vi "Autonomous Independent.vi"() -> ()   [LabVIEW 2020]
doc: "This VI is called when autonomous begins, and will automatically be terminated when autonomous ends. You can carry out timed or sensor driven robot movement independently without needing to return to the caller."
uses:
  <vilib>/Rock Robotics/Network Tables/NT Read String.vi
  <vilib>/Rock Robotics/WPI/Utilities/WPI_GetSetVariantRefNum.vi
  <vilib>/Rock Robotics/WPI/RobotDrive/WPI_RobotDriveArcadeDrive_Standard(NoSaturation).vi
  <vilib>/Rock Robotics/Network Tables/NT Write Numeric Array.vi
panel:
  out "Current Movement, for debugging":T1 {"Y Joystick Value" scale=1.0..-1.0; "X Joystick Value" scale=-1.0..1.0}
  in  "Array of robot movements":T2(array[cluster])=[{"X Joystick Value"=0.39393939393939403, "Y Joystick Value"=0.0, "Delay (sec)"=1.0, "Movement Name"="turn"}, {"X Joystick Value"=-0.3737373737373737, "Y Joystick Value"=0.0, "Delay (sec)"=1.0, "Movement Name"="turn back"}] {"Y Joystick Value" scale=1.0..-1.0; "X Joystick Value" scale=-1.0..1.0}
  # "Be sure to right-click and choose Data Operations>>Make Current Value default if you want to save the array values with the VI"
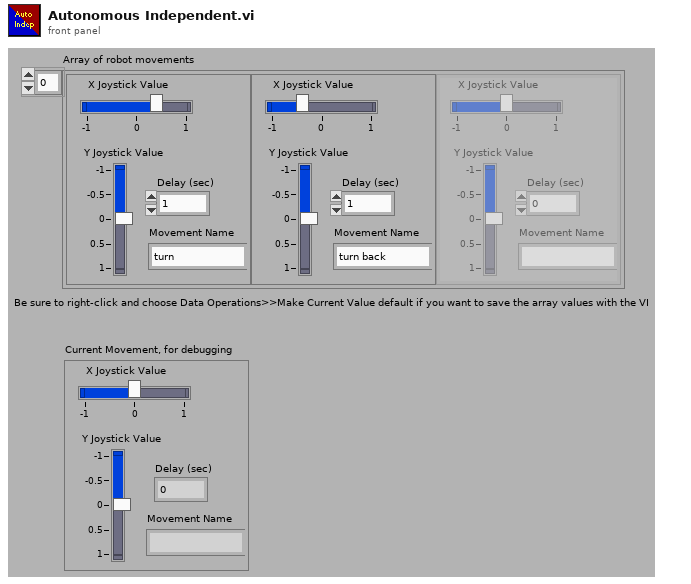
[diagram p1: front panel]
types:
  T1 = cluster{"X Joystick Value":dbl, "Y Joystick Value":dbl, "Delay (sec)":dbl, "Movement Name":string}
  T2 = cluster{"X Joystick Value":dbl, "Y Joystick Value":dbl, "Delay (sec)":dbl, "Movement Name":string}[]
  T3 = typedef "WPI_RobotDriveDevRef.ctl" = cluster{"DevStatus":errorcluster, "Motors[]":T4[], "Square Inputs":bool, "Max Output":dbl}
  T4 = typedef "WPI_MotorControlDeviceRef.ctl" = cluster{"DeviceStatus":errorcluster, "Type":T5, "PWM":cluster{"PWM Channel":T6, "DeadBand":T7}, "CAN":cluster{"Device Number":u8, "SetOutput VI Ref":variant, "GetOutput VI Ref":variant, "Enable VI Ref":variant, "Disable VI Ref":variant, "Data":variant}, "Invert":bool, "DIO PWM":cluster{"PWM \"Enable\" Channel":T6, "DIOChannel":T8, "PWM Rate":dbl}}
  T5 = typedef "WPI_MotorControlType.ctl" = enum16{"PWM", "CAN", "DIO PWM"}
  T6 = typedef "FPGA_DIOPWMChannel.ctl" = enum8{"PWM 0", "PWM 1", "PWM 2", "PWM 3", "PWM 4", "PWM 5", "PWM 6", "PWM 7", "PWM 8", "PWM 9", "PWM MXP 0", "PWM MXP 1", "PWM MXP 2", "PWM MXP 3", "PWM MXP 4", "PWM MXP 5", "PWM MXP 6", "PWM MXP 7", "PWM MXP 8", "PWM MXP 9", "Invalid"}
  T7 = typedef "WPI_PWMDeadband.ctl" = cluster{"Name":string, "maxPositivePwm":i32, "minPositivePwm":i32, "centerPwm":i32, "maxNegativePwm":i32, "minNegativePwm":i32, "angularRange":u16}
  T8 = typedef "FPGA_DIOChannel.ctl" = enum8{"DIO 0", "DIO 1", "DIO 2", "DIO 3", "DIO 4", "DIO 5", "DIO 6", "DIO 7", "DIO 8", "DIO 9", "DIO MXP 0", "DIO MXP 1", "DIO MXP 2", "DIO MXP 3", "DIO MXP 4", "DIO MXP 5", "DIO MXP 6", "DIO MXP 7", "DIO MXP 8", "DIO MXP 9", "DIO MXP 10", "DIO MXP 11", "DIO MXP 12", "DIO MXP 13", "DIO MXP 14", "DIO MXP 15", "SPI Port CS1", "SPI Port CS2", "SPI Port CS3", "SPI Port MISO", "SPI Port MOSI", "Invalid"}
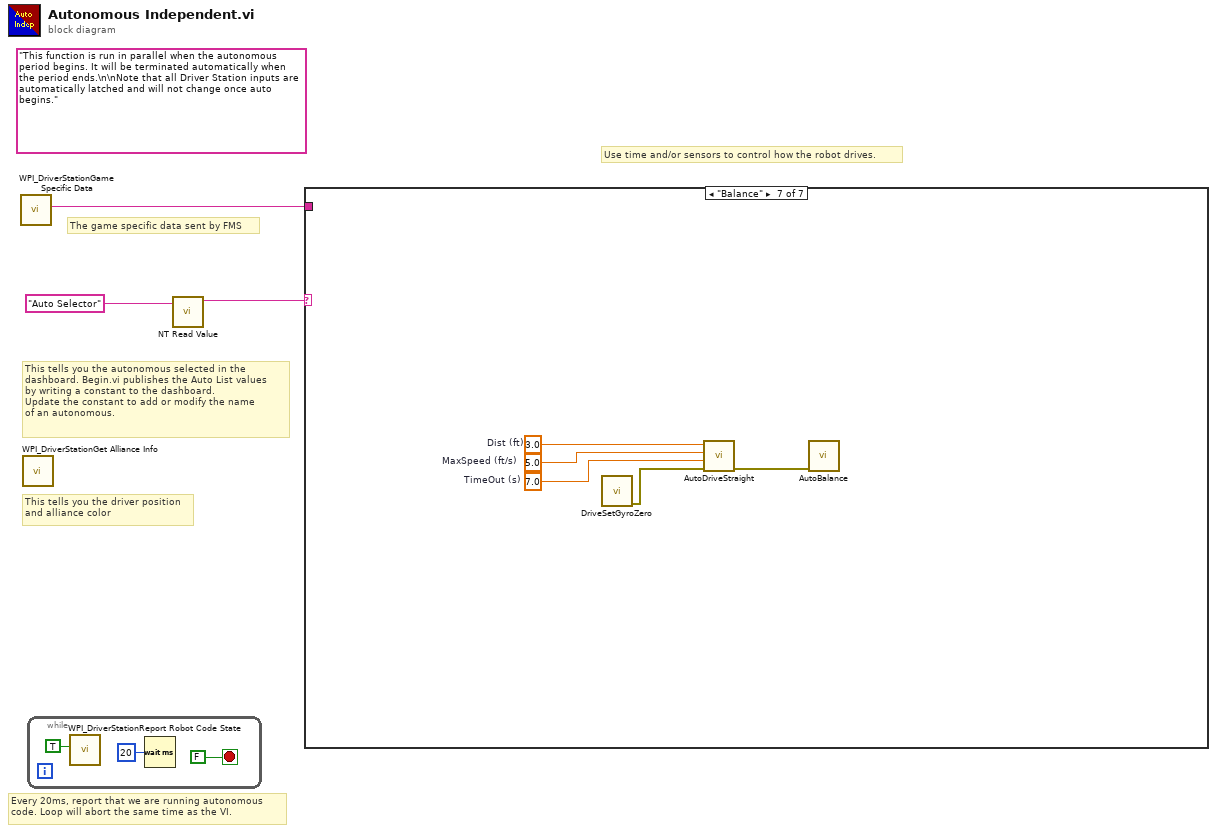
[diagram p0: block diagram]
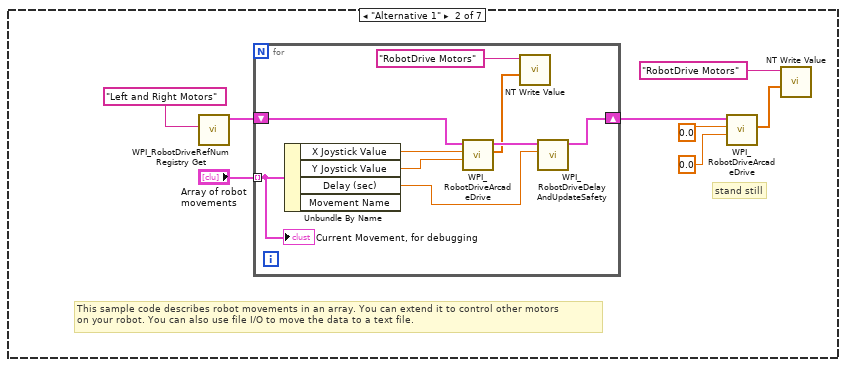
[diagram p3: hidden frame]
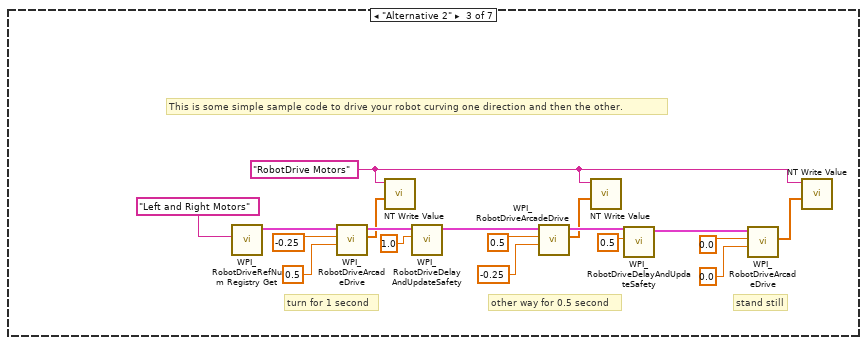
[diagram p4: hidden frame]
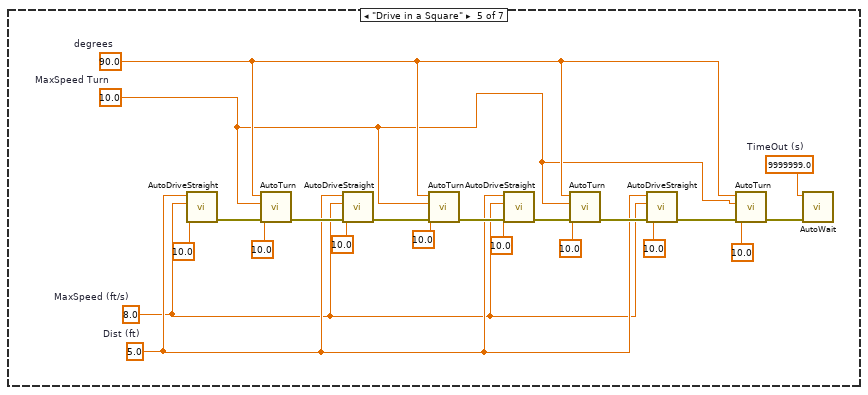
[diagram p6: hidden frame]
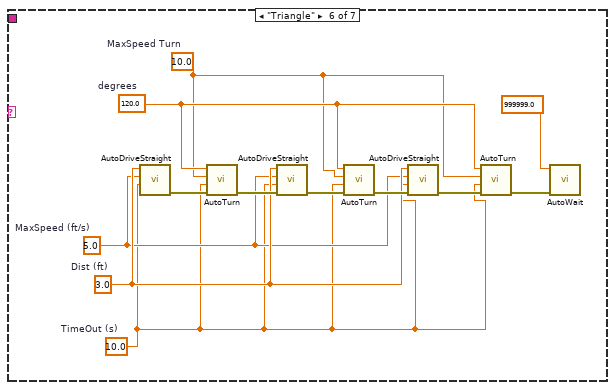
[diagram p7: hidden frame]
diagram:
  (unwired) "This function is run in parallel when the autonomous period begins. It will be terminated automatically when the period ends.\n\nNote that all Driver Station inputs are automatically latched and will not change once auto begins."
  # "The game specific data sent by FMS"
  # "This tells you the autonomous selected in the \ndashboard. Begin.vi publishes the Auto List values\nby writing a constant to the dashboard.\nUpdate the constant to add or modify the name\nof an autonomous."
  # "Every 20ms, report that we are running autonomous\ncode. Loop will abort the same time as the VI."
  # "Use time and/or sensors to control how the robot drives."
  # "This tells you the driver position\nand alliance color"
  n1 = call <vilib>:"WPI_DriverStationGame Specific Data.vi"() -> ("Game Specific Data"=w1:string)  [unwired: 11 in]
  n2 = call <vilib>:"WPI_DriverStationGet Alliance Info.vi"() -> ()  [unwired: 12 out]
  n3 = while {
    stop <- FALSE stop-if-true
    n4 = call <vilib>:"WPI_DriverStationReport Robot Code State.vi"("Autonomous"=TRUE) -> ()  [unwired: 10 in, 1 out]
    n5 = Wait (ms)(milliseconds to wait=u32 20) -> ()  [unwired: 1 out]
  }
  n6 = call-poly <vilib>:"NT Read Value.vi"("name"="Auto Selector" ("Name")) -> ("value"=w2:string)  [unwired: 8 in, 2 out]
  n7 = case shown="\"Balance\"" w2 {
    tunnel: w1 -> [_ _ _ _ _ _ _]
    frame Default {
      # "You can put your main auto here, or you can right-click on the case and make any\nother frame be the default case."
      # "This is the frame that will execute if no selection is made, or if it is not recognized"
    }
    frame "Alternative 1" {
      # "stand still"
      # "This sample code describes robot movements in an array. You can extend it to control other motors\non your robot. You can also use file I/O to move the data to a text file."
      n8 = call <vilib>:"WPI_RobotDriveRefNum Registry Get.vi"("refnum name"="Left and Right Motors") -> ("RobotDriveDevRef"=w13:T3)  [unwired: 1 in, 9 out]
      n9 = for {
        shift-right: [w21] -> w8
        shift-left: w13 -> [w22]
        tunnel: "Array of robot movements" -> [w17] mode=indexing
        n10 = Unbundle By Name(w17) -> ("X Joystick Value"=w20:dbl, "Y Joystick Value"=w19:dbl, "Delay (sec)"=w18:dbl)  [unwired: 1 out]
        n11 = call-poly <vilib>:"WPI_RobotDriveArcadeDrive.vi"("Y axis value"=w19, "X axis value"=w20, "RobotDriveDevRef"=w22) -> ("Motor Values"=w15:dbl[], "RobotDriveDevRef"=w23:T3)  [unwired: 1 in, 6 out]
        n12 = call-poly <vilib>:"NT Write Value.vi"("value"=w15, "name"="RobotDrive Motors" ("Name")) -> ()  [unwired: 9 in, 1 out]
        n13 = call <vilib>:"WPI_RobotDriveDelayAndUpdateSafety.vi"("Delay (s)"=w18, "RobotDriveDevRef"=w23) -> ("RobotDriveDevRef 2"=w21:T3)  [unwired: 8 in, 1 out]
        "Current Movement, for debugging" <- w17
      }
      n14 = call-poly <vilib>:"WPI_RobotDriveArcadeDrive.vi"("Y axis value"=0.0 ("X axis value"), "X axis value"=0.0, "RobotDriveDevRef"=w8) -> ("Motor Values"=w11:dbl[])  [unwired: 1 in, 7 out]
      n15 = call-poly <vilib>:"NT Write Value.vi"("value"=w11, "name"="RobotDrive Motors" ("Name")) -> ()  [unwired: 9 in, 1 out]
    }
    frame "Alternative 2" {
      w25 = "RobotDrive Motors" ("Name")
      # "This is some simple sample code to drive your robot curving one direction and then the other."
      # "stand still"
      # "other way for 0.5 second"
      # "turn for 1 second"
      n16 = call <vilib>:"WPI_RobotDriveRefNum Registry Get.vi"("refnum name"="Left and Right Motors") -> ("RobotDriveDevRef"=w41:T3)  [unwired: 1 in, 9 out]
      n17 = call-poly <vilib>:"WPI_RobotDriveArcadeDrive.vi"("Y axis value"=0.5 ("X axis value"), "X axis value"=-0.25, "RobotDriveDevRef"=w41) -> ("Motor Values"=w24:dbl[], "RobotDriveDevRef"=w34:T3)  [unwired: 1 in, 6 out]
      n18 = call-poly <vilib>:"NT Write Value.vi"("value"=w24, "name"=w25) -> ()  [unwired: 9 in, 1 out]
      n19 = call <vilib>:"WPI_RobotDriveDelayAndUpdateSafety.vi"("Delay (s)"=1.0, "RobotDriveDevRef"=w34) -> ("RobotDriveDevRef 2"=w35:T3)  [unwired: 8 in, 1 out]
      n20 = call-poly <vilib>:"WPI_RobotDriveArcadeDrive.vi"("Y axis value"=-0.25 ("X axis value"), "X axis value"=0.5, "RobotDriveDevRef"=w35) -> ("Motor Values"=w26:dbl[], "RobotDriveDevRef"=w36:T3)  [unwired: 1 in, 6 out]
      n21 = call-poly <vilib>:"NT Write Value.vi"("value"=w26, "name"=w25) -> ()  [unwired: 9 in, 1 out]
      n22 = call <vilib>:"WPI_RobotDriveDelayAndUpdateSafety.vi"("Delay (s)"=0.5, "RobotDriveDevRef"=w36) -> ("RobotDriveDevRef 2"=w37:T3)  [unwired: 8 in, 1 out]
      n23 = call-poly <vilib>:"WPI_RobotDriveArcadeDrive.vi"("Y axis value"=0.0 ("X axis value"), "X axis value"=0.0, "RobotDriveDevRef"=w37) -> ("Motor Values"=w27:dbl[])  [unwired: 1 in, 7 out]
      n24 = call-poly <vilib>:"NT Write Value.vi"("value"=w27, "name"=w25) -> ()  [unwired: 9 in, 1 out]
    }
    frame "Your Turn" {
    }
    frame "Drive in a Square" {
      w50 = 10.0  # MaxSpeed Turn
      w51 = 9999999.0  # TimeOut (s)
      w52 = 90.0  # degrees
      w53 = 8.0  # MaxSpeed (ft/s)
      w54 = 5.0  # Dist (ft)
      n25 = call "AutoDriveStraight.vi"("TimeOut (s)"=10.0, "MaxSpeed (ft/s)"=w53, "Dist (ft)"=w54) -> ("error out"=w55:errorcluster)  [unwired: 8 in]
      n26 = call "AutoTurn.vi"("error in (no error)"=w55, "TimeOut (s)"=10.0, "MaxSpeed (ft/s)"=w50, "degrees"=w52) -> ("error out"=w56:errorcluster)  [unwired: 7 in]
      n27 = call "AutoDriveStraight.vi"("error in (no error)"=w56, "TimeOut (s)"=10.0, "MaxSpeed (ft/s)"=w53, "Dist (ft)"=w54) -> ("error out"=w57:errorcluster)  [unwired: 7 in]
      n28 = call "AutoTurn.vi"("error in (no error)"=w57, "TimeOut (s)"=10.0, "MaxSpeed (ft/s)"=w50, "degrees"=w52) -> ("error out"=w58:errorcluster)  [unwired: 7 in]
      n29 = call "AutoDriveStraight.vi"("error in (no error)"=w58, "TimeOut (s)"=10.0, "MaxSpeed (ft/s)"=w53, "Dist (ft)"=w54) -> ("error out"=w59:errorcluster)  [unwired: 7 in]
      n30 = call "AutoTurn.vi"("error in (no error)"=w59, "TimeOut (s)"=10.0, "MaxSpeed (ft/s)"=w50, "degrees"=w52) -> ("error out"=w60:errorcluster)  [unwired: 7 in]
      n31 = call "AutoDriveStraight.vi"("error in (no error)"=w60, "TimeOut (s)"=10.0, "MaxSpeed (ft/s)"=w53, "Dist (ft)"=w54) -> ("error out"=w61:errorcluster)  [unwired: 7 in]
      n32 = call "AutoTurn.vi"("error in (no error)"=w61, "TimeOut (s)"=10.0, "MaxSpeed (ft/s)"=w50, "degrees"=w52) -> ("error out"=w62:errorcluster)  [unwired: 7 in]
      n33 = call "AutoWait.vi"("error in (no error)"=w62, "TimeOut (s)"=w51) -> ()  [unwired: 9 in, 1 out]
    }
    frame "Triangle" {
      w64 = 10.0  # TimeOut (s)
      w65 = 10.0  # MaxSpeed Turn
      w66 = 5.0  # MaxSpeed (ft/s)
      w67 = 120.0  # degrees
      w68 = 3.0  # Dist (ft)
      n34 = call "AutoDriveStraight.vi"("TimeOut (s)"=w64, "MaxSpeed (ft/s)"=w66, "Dist (ft)"=w68) -> ("error out"=w74:errorcluster)  [unwired: 8 in]
      n35 = call "AutoTurn.vi"("error in (no error)"=w74, "TimeOut (s)"=w64, "MaxSpeed (ft/s)"=w65, "degrees"=w67) -> ("error out"=w73:errorcluster)  [unwired: 7 in]
      n36 = call "AutoDriveStraight.vi"("error in (no error)"=w73, "TimeOut (s)"=w64, "MaxSpeed (ft/s)"=w66, "Dist (ft)"=w68) -> ("error out"=w72:errorcluster)  [unwired: 7 in]
      n37 = call "AutoTurn.vi"("error in (no error)"=w72, "TimeOut (s)"=w64, "MaxSpeed (ft/s)"=w65, "degrees"=w67) -> ("error out"=w71:errorcluster)  [unwired: 7 in]
      n38 = call "AutoDriveStraight.vi"("error in (no error)"=w71, "TimeOut (s)"=w64, "MaxSpeed (ft/s)"=w66, "Dist (ft)"=w68) -> ("error out"=w70:errorcluster)  [unwired: 7 in]
      n39 = call "AutoTurn.vi"("error in (no error)"=w70, "TimeOut (s)"=w64, "MaxSpeed (ft/s)"=w65, "degrees"=w67) -> ("error out"=w69:errorcluster)  [unwired: 7 in]
      n40 = call "AutoWait.vi"("error in (no error)"=w69, "TimeOut (s)"=999999.0) -> ()  [unwired: 9 in, 1 out]
    }
    frame "Balance" {
      w78 = 7.0  # TimeOut (s)
      w77 = 5.0  # MaxSpeed (ft/s)
      w79 = 3.0  # Dist (ft)
      n41 = call "DriveSetGyroZero.vi"() -> ("error out"=w75:errorcluster)  [unwired: 11 in]
      n42 = call "AutoDriveStraight.vi"("error in (no error)"=w75, "TimeOut (s)"=w78, "MaxSpeed (ft/s)"=w77, "Dist (ft)"=w79) -> ("error out"=w76:errorcluster)  [unwired: 7 in]
      n43 = call "AutoBalance.vi"("error in (no error)"=w76) -> ()  [unwired: 10 in, 1 out]
    }
  }
